vi "Save General Data(2).vi"(6 "Error In":errorcluster, 9 "Data Cluster":T1={"Message"="", "Homed?"=FALSE, "NextState"=enum."Timeout", "G.Load"=0.0, "G.Position"=0.0, "Load#"=0, "[G.Loads]"=[], "[TotalLoads]"=[], "[Errors]"=[], "ZeroWait"=0, "Results"=[], "DwellWait"=FALSE, "Test Result"=FALSE, "[CondyleLoads]"=[], "[Max]"=[], "[Min]"=[], "Valid String?"=FALSE, "ScanTime"=timestamp(0 s since 1904-01-01), "ScannedString"="", "LabelDevID"=0, "MfgDate"=timestamp(0 s since 1904-01-01), "[EEPROM Cmds]"=[], "[CalData]"=[], "[A/Ds]"=[], "[A/Dmax]"=[], "[A/Dmin]"=[], "BattMax"=0.0, "BattMin"=0.0, "DwellTime"=0, "PendingDeviceType"="", "Zero G.load"=0.0, "GAINC Value"="", "Programming Step"=enum."Load EEPROM", "Front Panel Program?"=FALSE, "Final Program?"=FALSE, "PCB Score"=100, "AssyScore"=100, "Pass/Fail #"="", "Result String"="", "Programming Mode"=enum."Initial Program", "Angle Test Step"=enum."Initialize", "Accel Values"=[], "Shutdown Counter"=0, "V1"=0, "V2"=5, "V3"=0, "V4"=0, "EEPROM Data"=[], "Counter"=0, "Page#"=0, "Timer"=timestamp(0 s since 1904-01-01), "Use Mark10?"=FALSE, "Eng-Result#"=0, "DUT Serial #"=0, "Scroll Message?"=FALSE, "Clear Message"=FALSE, "Batt Test Step "=enum."Initialize", "RXTX Window Found?"=FALSE, "Shutdown First Call?"=FALSE, "A2 Delay (msec)"=500, "Support Script"={"Script #"="", "Script Revision"="", "[OEMs]"=[], "[[DeviceTypes]]"=[], "[[DeviceTypesVals]]"=[], "[[List of Errors]]"=[], "Default GAINC"="", "[[ASICtrims]]"=[], "ID For Echo"="", "Condyle A CalFactor"=100, "Condyle B CalFactor"=100, "[OEMs Prefix]"=[], "Packet ID 18"="", "[[Force Table Load Test]]"=[], "[[Force Table AccurTest]]"=[]}, "Serial Table"={"Serial File Path"=path "", "[[Serial Lookup Table]]"=[], "Serial Device Info"=[], "Valid Serial?"=FALSE}, "Target Information"={"Target Brand"="", "Target DeviceType"="", "Target Serial#"=100, "Target Lot#"=0, "Target DevID"=0, "Target Channel"=5}, "Operator"="", "COM Port"="", "Config Path"=path "", "Tx Array"=[], "DUT Parameters"={"Channel"=0, "DeviceID"=0, "Script Rev"=0, "Month"=0, "Day"=0, "Year"=0, "Lot#"=0, "V1"=0, "V2"=0, "V3"=0, "V4"=0, "MFG"=0, "Cal FactorA"=0, "Cal FactorB"=0, "ASICtrim"=[], "TmpChan"=0, "GAINC"="", "Brand"="", "Device"="", "Serial #"=0, "Batt310"=0, "Batt 280"=0}, "FTS Main?"=FALSE, "Loading"={"[Forces]"=[], "[Dwell]"=[], "Loading Step"=enum."Initialize Test"}, "Software Version"="", "Correction Factor"="", "Second Load Test"=FALSE, "Acc Loads"=[], "Mark10 Config"={"H2S%"=[80.0, 85.0, 90.0, 95.0, 100.0], "H2S Speed"=[12.0, 8.0, 6.0, 4.0, 2.0], "H to S"=2.0, "Home Speed"=1.0, "LoadWin"=0.0, "Load Speed"=0.0, "PID"={"Kp"=0.04, "Kd"=0.005001, "Ki"=2.9999999999999923e-05}}, "Channels"={"Transceiver Ch"=5, "Operating Ch"=5, "Start Ch"=0}} {"Mark10 Config"."PID"."Ki" min=0.0 max=200.0 format="%.6f"; "Mark10 Config"."PID"."Kd" min=0.0 max=200.0 format="%.6f"; "Mark10 Config"."PID"."Kp" min=0.0 max=200.0 format="%.6f"; "DUT Parameters"."ASICtrim" format="%02x"}) -> (0 "error out":errorcluster, 3 "Data Out":T1={"Message"="", "Homed?"=FALSE, "NextState"=enum."Timeout", "G.Load"=0.0, "G.Position"=0.0, "Load#"=0, "[G.Loads]"=[], "[TotalLoads]"=[], "[Errors]"=[], "ZeroWait"=0, "Results"=[], "DwellWait"=FALSE, "Test Result"=FALSE, "[CondyleLoads]"=[], "[Max]"=[], "[Min]"=[], "Valid String?"=FALSE, "ScanTime"=timestamp(0 s since 1904-01-01), "ScannedString"="", "LabelDevID"=0, "MfgDate"=timestamp(0 s since 1904-01-01), "[EEPROM Cmds]"=[], "[CalData]"=[], "[A/Ds]"=[], "[A/Dmax]"=[], "[A/Dmin]"=[], "BattMax"=0.0, "BattMin"=0.0, "DwellTime"=0, "PendingDeviceType"="", "Zero G.load"=0.0, "GAINC Value"="", "Programming Step"=enum."Load EEPROM", "Front Panel Program?"=FALSE, "Final Program?"=FALSE, "PCB Score"=100, "AssyScore"=100, "Pass/Fail #"="", "Result String"="", "Programming Mode"=enum."Initial Program", "Angle Test Step"=enum."Initialize", "Accel Values"=[], "Shutdown Counter"=0, "V1"=0, "V2"=5, "V3"=0, "V4"=0, "EEPROM Data"=[], "Counter"=0, "Page#"=0, "Timer"=timestamp(0 s since 1904-01-01), "Use Mark10?"=FALSE, "Eng-Result#"=0, "DUT Serial #"=0, "Scroll Message?"=FALSE, "Clear Message"=FALSE, "Batt Test Step "=enum."Initialize", "RXTX Window Found?"=FALSE, "Shutdown First Call?"=FALSE, "A2 Delay (msec)"=500, "Support Script"={"Script #"="", "Script Revision"="", "[OEMs]"=[], "[[DeviceTypes]]"=[], "[[DeviceTypesVals]]"=[], "[[List of Errors]]"=[], "Default GAINC"="", "[[ASICtrims]]"=[], "ID For Echo"="", "Condyle A CalFactor"=100, "Condyle B CalFactor"=100, "[OEMs Prefix]"=[], "Packet ID 18"="", "[[Force Table Load Test]]"=[], "[[Force Table AccurTest]]"=[]}, "Serial Table"={"Serial File Path"=path "", "[[Serial Lookup Table]]"=[], "Serial Device Info"=[], "Valid Serial?"=FALSE}, "Target Information"={"Target Brand"="", "Target DeviceType"="", "Target Serial#"=100, "Target Lot#"=0, "Target DevID"=0, "Target Channel"=5}, "Operator"="", "COM Port"="", "Config Path"=path "", "Tx Array"=[], "DUT Parameters"={"Channel"=0, "DeviceID"=0, "Script Rev"=0, "Month"=0, "Day"=0, "Year"=0, "Lot#"=0, "V1"=0, "V2"=0, "V3"=0, "V4"=0, "MFG"=0, "Cal FactorA"=0, "Cal FactorB"=0, "ASICtrim"=[], "TmpChan"=0, "GAINC"="", "Brand"="", "Device"="", "Serial #"=0, "Batt310"=0, "Batt 280"=0}, "FTS Main?"=FALSE, "Loading"={"[Forces]"=[], "[Dwell]"=[], "Loading Step"=enum."Initialize Test"}, "Software Version"="", "Correction Factor"="", "Second Load Test"=FALSE, "Acc Loads"=[], "Mark10 Config"={"H2S%"=[80.0, 85.0, 90.0, 95.0, 100.0], "H2S Speed"=[12.0, 8.0, 6.0, 4.0, 2.0], "H to S"=2.0, "Home Speed"=1.0, "LoadWin"=0.0, "Load Speed"=0.0, "PID"={"Kp"=0.04, "Kd"=0.005001, "Ki"=2.9999999999999923e-05}}, "Channels"={"Transceiver Ch"=5, "Operating Ch"=5, "Start Ch"=0}} {"Mark10 Config"."PID"."Ki" min=0.0 max=200.0 format="%.6f"; "Mark10 Config"."PID"."Kd" min=0.0 max=200.0 format="%.6f"; "Mark10 Config"."PID"."Kp" min=0.0 max=200.0 format="%.6f"; "DUT Parameters"."ASICtrim" format="%02x"})   [LabVIEW 2013]
uses:
  Controls/LocalVars.ctl
  Controls/Gen2 FT states.ctl
  Controls/Iniial Device Programming.ctl
  SubVI/ProgramStageControl.ctl
  Controls/Batt Cap Steps.ctl
  Controls/Support Script.ctl
  Controls/Serial Table.ctl
  Controls/Device Information.ctl
  Controls/InfoPacket.ctl
  Controls/Loading.ctl
  Controls/Load Step.ctl
  Controls/Mark10 Config.ctl
  Controls/PID parameters.ctl
  Controls/Channels.ctl
  <vilib>/Utility/NIReport.llb/NI_report.lvclass
  <vilib>/Utility/NIReport.llb/Excel/NI_Excel.lvclass
  <vilib>/addons/_office/NI_ReportGenerationToolkit.lvlib
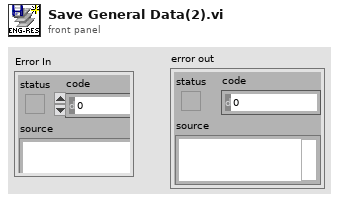
[diagram p1: front panel]
types:
  T1 = typedef "LocalVars.ctl" = cluster{"Message":string, "Homed?":bool, "NextState":T2, "G.Load":dbl, "G.Position":dbl, "Load#":i32, "[G.Loads]":dbl[], "[TotalLoads]":dbl[], "[Errors]":dbl[][], "ZeroWait":u32, "Results":dbl[], "DwellWait":bool, "Test Result":bool, "[CondyleLoads]":dbl[][], "[Max]":dbl[], "[Min]":dbl[], "Valid String?":bool, "ScanTime":timestamp, "ScannedString":string, "LabelDevID":u32, "MfgDate":timestamp, "[EEPROM Cmds]":u8[][], "[CalData]":u8[][], "[A/Ds]":dbl[][], "[A/Dmax]":dbl[], "[A/Dmin]":dbl[], "BattMax":dbl, "BattMin":dbl, "DwellTime":i32, "PendingDeviceType":string, "Zero G.load":dbl, "GAINC Value":string, "Programming Step":T3, "Front Panel Program?":bool, "Final Program?":bool, "PCB Score":i32, "AssyScore":i32, "Pass/Fail #":string, "Result String":string, "Programming Mode":T4, "Angle Test Step":enum16{"Initialize", "Get X", "Get Y", "Get Z", "Next Test"}, "Accel Values":dbl[][], "Shutdown Counter":u32, "V1":i32, "V2":i32, "V3":i32, "V4":i32, "EEPROM Data":i32[][], "Counter":i32, "Page#":i32, "Timer":timestamp, "Use Mark10?":bool, "Eng-Result#":u32, "DUT Serial #":i32, "Scroll Message?":bool, "Clear Message":bool, "Batt Test Step ":T5, "RXTX Window Found?":bool, "Shutdown First Call?":bool, "A2 Delay (msec)":i16, "Support Script":T6, "Serial Table":T7, "Target Information":T8, "Operator":string, "COM Port":string, "Config Path":path, "Tx Array":u8[], "DUT Parameters":T9, "FTS Main?":bool, "Loading":T10, "Software Version":string, "Correction Factor":string, "Second Load Test":bool, "Acc Loads":dbl[][], "Mark10 Config":T12, "Channels":T14}
  T2 = typedef "Gen2 FT states.ctl" = enum16{"---------SETUP-------", "Initialization", "Read Support Data", "Initialize Mark-10", "Initialize Transceiver", "------UTILITIES------", "Change DUT Channel", "Find RxTx Window", "Reset Device", "Scan Channels", "Read Serial Lookup", "Shutdown Device", "ESTOP", "--------USER---------", "Timeout", "-----PROGRAM-----", "Program Device", "------MARK10--------", "Go Home", "MoveUp", "MoveDown", "Goto Load", "Goto Position", "Stop Motor", "---------TESTS--------", "Start Test", "Angle Test", "Load Test", "Load Accuracy Test", "Battery Test", "------RESULTS-------", "End Test", "Display Result", "--------EXIT--------", "Exit"}
  T3 = typedef "Iniial Device Programming.ctl" = enum16{"Load EEPROM", "Send First A1", "Send EEPROM", "Send A1", "Check EEPROM Echo", "Verify transmission", "Programming Successful", "Programming Failed"}
  T4 = typedef "ProgramStageControl.ctl" = enum16{"Initial Program", "GainC", "Scales"}
  T5 = typedef "Batt Cap Steps.ctl" = enum16{"Initialize", "Collect 2.8 Volts", "Collect 3.1 Volts", "Check Results"}
  T6 = typedef "Support Script.ctl" = cluster{"Script #":string, "Script Revision":string, "[OEMs]":string[], "[[DeviceTypes]]":string[][], "[[DeviceTypesVals]]":u16[][], "[[List of Errors]]":string[][], "Default GAINC":string, "[[ASICtrims]]":u8[][], "ID For Echo":string, "Condyle A CalFactor":i32, "Condyle B CalFactor":i32, "[OEMs Prefix]":string[], "Packet ID 18":string, "[[Force Table Load Test]]":dbl[][], "[[Force Table AccurTest]]":dbl[][]}
  T7 = typedef "Serial Table.ctl" = cluster{"Serial File Path":path, "[[Serial Lookup Table]]":string[][], "Serial Device Info":string[], "Valid Serial?":bool}
  T8 = typedef "Device Information.ctl" = cluster{"Target Brand":string, "Target DeviceType":string, "Target Serial#":i32, "Target Lot#":u32, "Target DevID":u32, "Target Channel":u8}
  T9 = typedef "InfoPacket.ctl" = cluster{"Channel":u8, "DeviceID":u32, "Script Rev":u8, "Month":u8, "Day":u8, "Year":u8, "Lot#":u32, "V1":u16, "V2":u16, "V3":u16, "V4":u16, "MFG":u8, "Cal FactorA":u8, "Cal FactorB":u8, "ASICtrim":u8[], "TmpChan":u8, "GAINC":string, "Brand":string, "Device":string, "Serial #":u64, "Batt310":u16, "Batt 280":u16}
  T10 = typedef "Loading.ctl" = cluster{"[Forces]":dbl[], "[Dwell]":dbl[], "Loading Step":T11}
  T11 = typedef "Load Step.ctl" = enum16{"Initialize Test", "Go Home", "Detect Dev Surface", "Wait to zero Device", "Zero Device", "Do Test", "Test Result"}
  T12 = typedef "Mark10 Config.ctl" = cluster{"H2S%":dbl[], "H2S Speed":dbl[], "H to S":dbl, "Home Speed":dbl, "LoadWin":dbl, "Load Speed":dbl, "PID":T13}
  T13 = typedef "PID parameters.ctl" = cluster{"Kp":dbl, "Kd":dbl, "Ki":dbl}
  T14 = typedef "Channels.ctl" = cluster{"Transceiver Ch":u8, "Operating Ch":u8, "Start Ch":u8}
  T15 = enum16{"maximized", "minimized", "normal", "no change"}
  T16 = enum16{"Standard Report", "HTML", "Word", "Excel"}
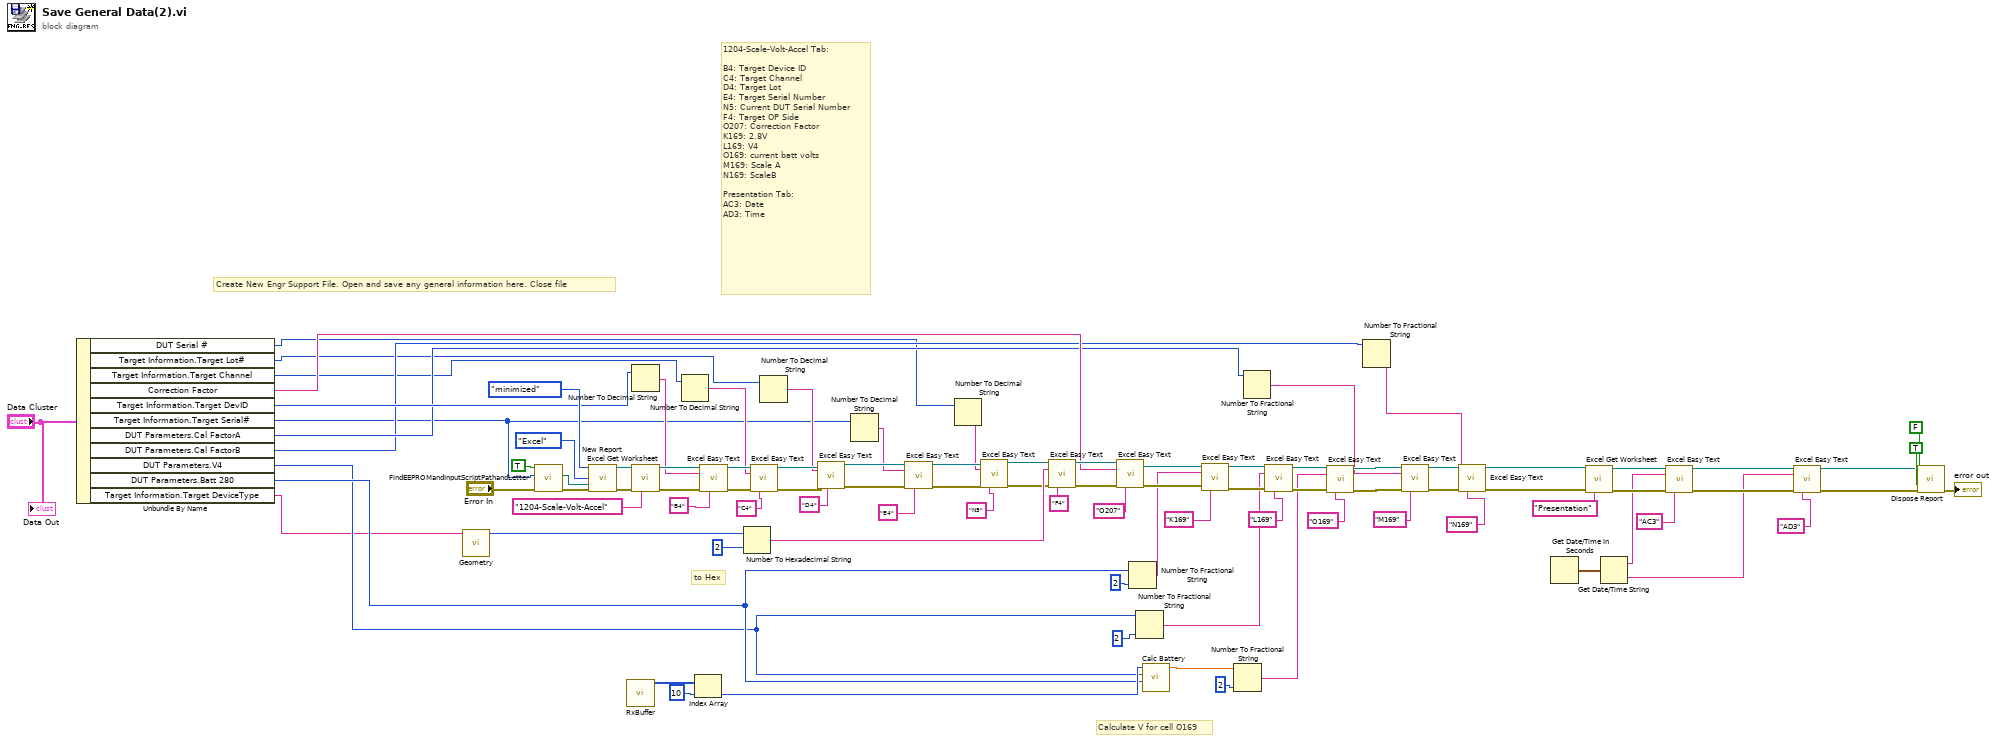
[diagram p0: block diagram]
diagram:
  # "1204-Scale-Volt-Accel Tab:\n\nB4: Target Device ID\nC4: Target Channel\nD4: Target Lot\nE4: Target Serial Number\nN5: Current DUT Serial Number\nF4: Target OP Side\nO207: Correction Factor\nK169: 2.8V\nL169: V4\nO169: current batt volts\nM169: Scale A\nN169: ScaleB\n\nPresentation Tab:\nAC3: Date\nAD3: Time"
  # "to Hex"
  # "Calculate V for cell O169"
  # "Create New Engr Support File. Open and save any general information here. Close file"
  n1 = Unbundle By Name("Data Cluster") -> ("DUT Serial #"=w2:i32, "Target Information.Target Lot#"=w15:u32, "Target Information.Target Channel"=w11:u8, "Correction Factor"=w60:string, "Target Information.Target DevID"=w78:u32, "Target Information.Target Serial#"=w9:i32, "DUT Parameters.Cal FactorA"=w30:u8, "DUT Parameters.Cal FactorB"=w28:u8, "DUT Parameters.V4"=w45:u16, "DUT Parameters.Batt 280"=w51:u16, "Target Information.Target DeviceType"=w24:string)
  n2 = call "Geometry.vi"("DeviceType"=w24) -> ("MFG"=w23:i32)  [unwired: 10 in]
  n3 = call "FindEEPROMandInputScriptPathandLetter.vi"("Error In"="Error In", "Eng-Result #"=w9, "Create New Engr Results? (F)"=TRUE) -> ("Error Out"=w83:errorcluster, "Engr Result Path"=w94:path)  [unwired: 4 in, 1 out]
  n4 = call <vilib>:"New Report.vi"("window state (normal)"=T15."minimized", "report type"=T16."Excel", "template (empty)"=w94, "error in (no error)"=w83) -> ("report out"=w81:refnum<class "NI_report.lvclass">, "error out"=w82:errorcluster)  [unwired: 10 in]
  n5 = call "RxBuffer.vi"() -> ("RxData Out"=w56:u16[])  [unwired: 9 in, 10 out]
  n6 = Number To Decimal String(number=w78) -> (decimal integer string=w85:string)  [unwired: 1 in]
  n7 = call <vilib>:"Excel Get Worksheet.vi"("report in"=w81, "error in (no error)"=w82, "name (\"\")"="1204-Scale-Volt-Accel" ("name (\"\")")) -> ("report out"=w89:refnum<class "NI_report.lvclass">, "error out"=w88:errorcluster)  [unwired: 11 in]
  n8 = Number To Decimal String(number=w11) -> (decimal integer string=w19:string)  [unwired: 1 in]
  n9 = Index Array(array=w56, index=10) -> (element=w55:u16)
  n10 = call <vilib>:"Excel Easy Text.vi"("report in"=w89, "text"=w85, "error in (no error)"=w88, "name (\"\")"="B4" ("name (\"\")")) -> ("report out"=w22:refnum<class "NI_report.lvclass">, "error out"=w21:errorcluster)  [unwired: 7 in, 3 out]
  n11 = Number To Hexadecimal String(1:2, 2:w23) -> (0:w76:string)
  n12 = call <vilib>:"Excel Easy Text.vi"("report in"=w22, "text"=w19, "error in (no error)"=w21, "name (\"\")"="C4" ("name (\"\")")) -> ("report out"=w17:refnum<class "NI_report.lvclass">, "error out"=w18:errorcluster)  [unwired: 7 in, 3 out]
  n13 = Number To Decimal String(number=w15) -> (decimal integer string=w14:string)  [unwired: 1 in]
  n14 = call <vilib>:"Excel Easy Text.vi"("report in"=w17, "text"=w14, "error in (no error)"=w18, "name (\"\")"="D4" ("name (\"\")")) -> ("report out"=w13:refnum<class "NI_report.lvclass">, "error out"=w12:errorcluster)  [unwired: 7 in, 3 out]
  n15 = Number To Decimal String(number=w9) -> (decimal integer string=w8:string)  [unwired: 1 in]
  n16 = call <vilib>:"Excel Easy Text.vi"("report in"=w13, "text"=w8, "error in (no error)"=w12, "name (\"\")"="E4" ("name (\"\")")) -> ("report out"=w7:refnum<class "NI_report.lvclass">, "error out"=w6:errorcluster)  [unwired: 7 in, 3 out]
  n17 = Number To Decimal String(number=w2) -> (decimal integer string=w1:string)  [unwired: 1 in]
  n18 = call <vilib>:"Excel Easy Text.vi"("report in"=w7, "text"=w1, "error in (no error)"=w6, "name (\"\")"="N5" ("name (\"\")")) -> ("report out"=w4:refnum<class "NI_report.lvclass">, "error out"=w3:errorcluster)  [unwired: 7 in, 3 out]
  n19 = call <vilib>:"Excel Easy Text.vi"("report in"=w4, "text"=w76, "error in (no error)"=w3, "name (\"\")"="F4" ("name (\"\")")) -> ("report out"=w61:refnum<class "NI_report.lvclass">, "error out"=w62:errorcluster)  [unwired: 7 in, 3 out]
  n20 = call <vilib>:"Excel Easy Text.vi"("report in"=w61, "text"=w60, "error in (no error)"=w62, "name (\"\")"="O207" ("name (\"\")")) -> ("report out"=w52:refnum<class "NI_report.lvclass">, "error out"=w53:errorcluster)  [unwired: 7 in, 3 out]
  n21 = Number To Fractional String(number=w51, precision (6)=i16 2 ("width (-)")) -> (F-format string=w49:string)  [unwired: 2 in]
  n22 = Number To Fractional String(number=w45, precision (6)=i16 2 ("width (-)")) -> (F-format string=w44:string)  [unwired: 2 in]
  n23 = call "Calc Battery.vi"("Batt 280"=w51, "Batt310"=w45, "AD"=w55) -> ("Batt Volt"=w39:dbl)  [unwired: 8 in]
  n24 = call <vilib>:"Excel Easy Text.vi"("report in"=w52, "text"=w49, "error in (no error)"=w53, "name (\"\")"="K169" ("name (\"\")")) -> ("report out"=w47:refnum<class "NI_report.lvclass">, "error out"=w48:errorcluster)  [unwired: 7 in, 3 out]
  n25 = Number To Fractional String(number=w39, precision (6)=i16 2 ("width (-)")) -> (F-format string=w37:string)  [unwired: 2 in]
  n26 = Number To Fractional String(number=w30) -> (F-format string=w29:string)  [unwired: 3 in]
  n27 = call <vilib>:"Excel Easy Text.vi"("report in"=w47, "text"=w44, "error in (no error)"=w48, "name (\"\")"="L169" ("name (\"\")")) -> ("report out"=w41:refnum<class "NI_report.lvclass">, "error out"=w40:errorcluster)  [unwired: 7 in, 3 out]
  n28 = call <vilib>:"Excel Easy Text.vi"("report in"=w41, "text"=w37, "error in (no error)"=w40, "name (\"\")"="O169" ("name (\"\")")) -> ("report out"=w36:refnum<class "NI_report.lvclass">, "error out"=w35:errorcluster)  [unwired: 7 in, 3 out]
  n29 = Number To Fractional String(number=w28) -> (F-format string=w27:string)  [unwired: 3 in]
  n30 = call <vilib>:"Excel Easy Text.vi"("report in"=w36, "text"=w29, "error in (no error)"=w35, "name (\"\")"="M169" ("name (\"\")")) -> ("report out"=w32:refnum<class "NI_report.lvclass">, "error out"=w33:errorcluster)  [unwired: 7 in, 3 out]
  n31 = call <vilib>:"Excel Easy Text.vi"("report in"=w32, "text"=w27, "error in (no error)"=w33, "name (\"\")"="N169" ("name (\"\")")) -> ("report out"=w26:refnum<class "NI_report.lvclass">, "error out"=w25:errorcluster)  [unwired: 7 in, 3 out]
  n32 = Get Date/Time In Seconds() -> (seconds since 1Jan1904=w68:timestamp)
  n33 = call <vilib>:"Excel Get Worksheet.vi"("report in"=w26, "error in (no error)"=w25, "name (\"\")"="Presentation" ("name (\"\")")) -> ("report out"=w73:refnum<class "NI_report.lvclass">, "error out"=w72:errorcluster)  [unwired: 11 in]
  n34 = Get Date/Time String(seconds (now)=w68) -> (date string=w67:string, time string=w66:string)  [unwired: 2 in]
  n35 = call <vilib>:"Excel Easy Text.vi"("report in"=w73, "text"=w67, "error in (no error)"=w72, "name (\"\")"="AC3" ("name (\"\")")) -> ("report out"=w65:refnum<class "NI_report.lvclass">, "error out"=w71:errorcluster)  [unwired: 7 in, 3 out]
  n36 = call <vilib>:"Excel Easy Text.vi"("report in"=w65, "text"=w66, "error in (no error)"=w71, "name (\"\")"="AD3" ("name (\"\")")) -> ("report out"=w64:refnum<class "NI_report.lvclass">, "error out"=w63:errorcluster)  [unwired: 7 in, 3 out]
  n37 = call-dynamic "Dispose Report.vi"("report in"=w64, "wait until printing completed? (T)"=FALSE, "save changes? (F)"=TRUE, "error in (no error)"=w63) -> ("error out"=→"error out":errorcluster)  [unwired: 11 in]
  "Data Out" <- "Data Cluster"
